vi "Actor Core.vi"(8 "error in":errorcluster, 11 "My Application":refnum<class "App Actor.lvclass">) -> (0 "error out":errorcluster, 3 "Actor out":refnum<class "Actor.lvclass">)   [LabVIEW 2024, in "App Actor.lvlib" / "App Actor.lvclass"]
doc: "This is Actor Core.vi, the main message handling loop for Actors. An actor usually just sits in this loop and processes messages as they arrive. Any error returned by the message Do.vi call will stop the loop, with error code 43 as the canonical signal to stop with no error sent to caller. Descendants may override that in Handle Error.vi."
uses:
  App Actor.lvclass
  C:/Program Files (x86)/National Instruments/LabVIEW 2024/vi.lib/ActorFramework/Actor/Actor.lvclass
  <vilib>/ActorFramework/Actor/Actor.lvclass
  HAL Interface Actor/HAL Interface Actor/HAL Interface Actor.lvclass
  DAQ Actor/DAQ Actor/DAQ Actor.lvclass
  <vilib>/ActorFramework/Actor/Actor.lvclass/Actor.ctl
  <vilib>/ActorFramework/Message Enqueuer/Message Enqueuer.lvclass/Message Enqueuer.ctl
  App Actor.lvclass/App Actor.ctl
  DAQ Actor/DAQ Actor Task Msg/DAQ Actor Task Msg.lvclass/DAQ Actor Task Msg.ctl
  HAL Interface Actor/HAL Interface Actor Task Msg/HAL Interface Actor Task Msg.lvclass/HAL Interface Actor Task Msg.ctl
  <vilib>/ActorFramework/Message Enqueuer/Init from Existing Queue.vi
  <vilib>/ActorFramework/Message Enqueuer/Enqueue.vi
  <vilib>/ActorFramework/Stop Msg/Stop Msg.lvclass
  C:/Program Files (x86)/National Instruments/LabVIEW 2024/vi.lib/ActorFramework/Message/Message.lvclass
  DAQ Actor/DAQ Actor Task Msg/DAQ Actor Task Msg.lvclass
  HAL Interface Actor/HAL Interface Actor Task Msg/HAL Interface Actor Task Msg.lvclass
  <vilib>/ActorFramework/Message Priority Queue/Priority Enqueue.vi
  <vilib>/ActorFramework/Message Enqueuer/Message Enqueuer.lvclass
panel:
  in  "stop signal":bool
  out "Event Log":string
  in  "Stop":bool
  in  "Message to DAQ Actor":bool
  in  "Message to HAL Interface Actor":bool
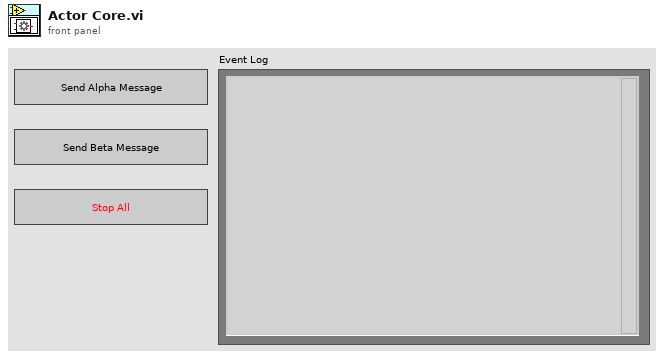
[diagram p1: front panel]
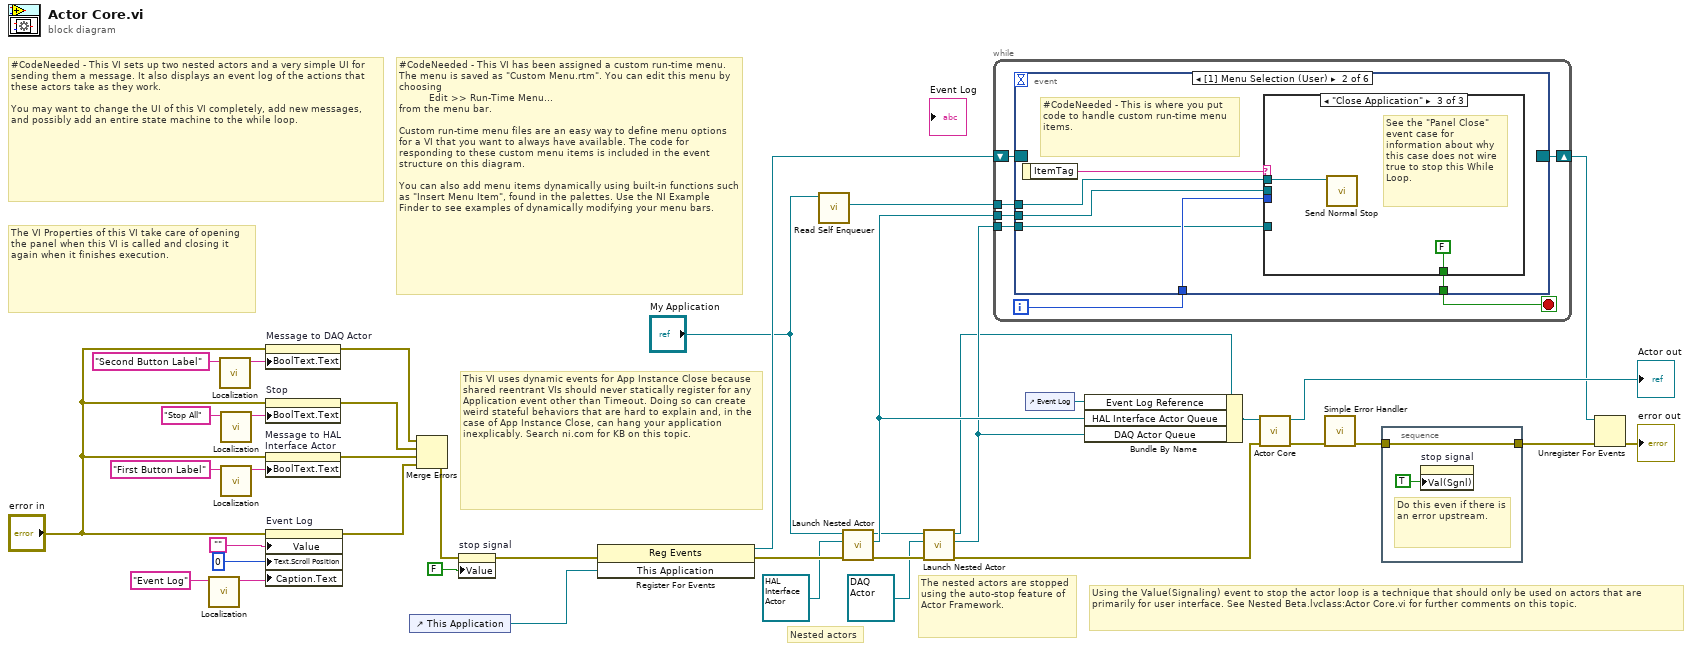
[diagram p0: block diagram]
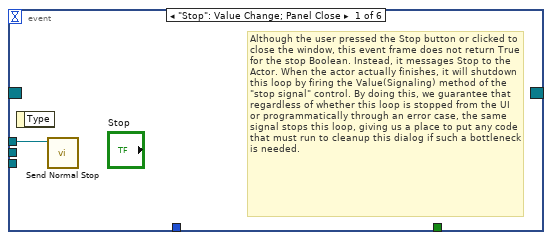
[diagram p2: hidden frame]
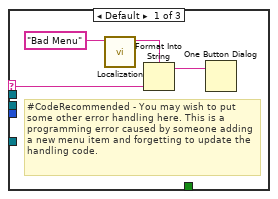
[diagram p3: hidden frame]
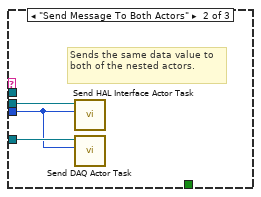
[diagram p4: hidden frame]
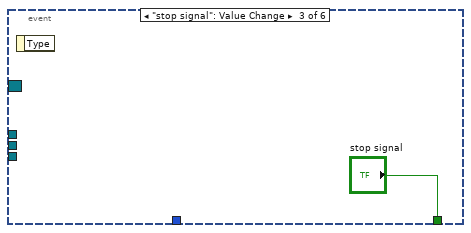
[diagram p5: hidden frame]
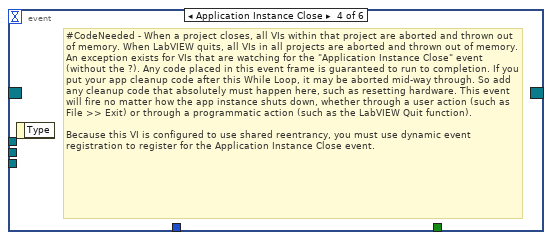
[diagram p6: hidden frame]
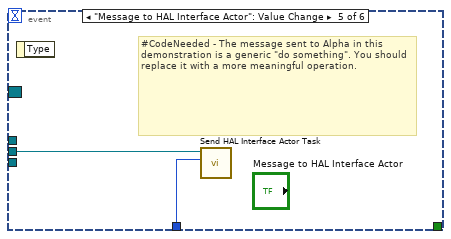
[diagram p7: hidden frame]
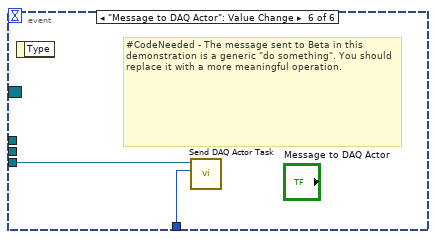
[diagram p8: hidden frame]
diagram:
  # "Nested actors"
  # "The nested actors are stopped using the auto-stop feature of Actor Framework."
  # "#CodeNeeded - This VI has been assigned a custom run-time menu. The menu is saved as \"Custom Menu.rtm\". You can edit this menu by choosing \n          Edit >> Run-Time Menu...\nfrom the menu bar.\n\nCustom run-time menu files are an easy way to define menu options for a VI that you want to always have available. The code for responding to these custom menu items is included in the event structure on this diagram.\n\nYou can also add menu items dynamically using built-in functions such as \"Insert Menu Item\", found in the palettes. Use the NI Example Finder to see examples of dynamically modifying your menu bars."
  # "This VI uses dynamic events for App Instance Close because shared reentrant VIs should never statically register for any Application event other than Timeout. Doing so can create weird stateful behaviors that are hard to explain and, in the case of App Instance Close, can hang your application inexplicably. Search ni.com for KB on this topic."
  # "The VI Properties of this VI take care of opening the panel when this VI is called and closing it again when it finishes execution."
  # "Using the Value(Signaling) event to stop the actor loop is a technique that should only be used on actors that are primarily for user interface. See Nested Beta.lvclass:Actor Core.vi for further comments on this topic."
  # "#CodeNeeded - This VI sets up two nested actors and a very simple UI for sending them a message. It also displays an event log of the actions that these actors take as they work. \n\nYou may want to change the UI of this VI completely, add new messages, and possibly add an entire state machine to the while loop."
  n1 = call "Localization.vi"("Unlocalized"="Event Log") -> ("Localized"=w26:string)  [unwired: 10 in]
  n2 = call "Localization.vi"("Unlocalized"="Second Button Label") -> ("Localized"=w20:string)  [unwired: 10 in]
  n3 = call "Localization.vi"("Unlocalized"="Stop All") -> ("Localized"=w22:string)  [unwired: 10 in]
  n4 = call "Localization.vi"("Unlocalized"="First Button Label") -> ("Localized"=w24:string)  [unwired: 10 in]
  n5 = property on="Message to DAQ Actor" class="Bool"(error in="error in", "BoolText.Text"=w20) -> (error out=w19:errorcluster)  [unwired: 1 in, 1 out]
  n6 = property on="Stop" class="Bool"(error in="error in", "BoolText.Text"=w22) -> (error out=w18:errorcluster)  [unwired: 1 in, 1 out]
  n7 = property on="Message to HAL Interface Actor" class="Bool"(error in="error in", "BoolText.Text"=w24) -> (error out=w17:errorcluster)  [unwired: 1 in, 1 out]
  n8 = property on="Event Log" class="Str"(error in="error in", "Value"="", "Text.Scroll Position"=u32 0, "Caption.Text"=w26) -> (error out=w16:errorcluster)  [unwired: 1 in, 1 out]
  n9 = control-ref of="This Application"() -> (w6:refnum<vi>)
  n10 = Merge Errors(w19, w18, w17, w16) -> (w15:errorcluster)
  n11 = property on="stop signal" class="Bool (strict)"(error in=w15, "Value"=FALSE ("stop")) -> (error out=w8:errorcluster)  [unwired: 1 in, 1 out]
  n12 = register-events(error in=w8, w6) -> (reference out=w12:refnum<event-registration>, error out=w7:errorcluster)  [unwired: 1 in]
  n13 = call <vilib>:"Read Self Enqueuer.vi"("Actor"="My Application") -> ("Self Enqueuer"=w34:refnum<class "Message Enqueuer.lvclass">)  [unwired: 10 in]
  n14 = call <vilib>:"Launch Nested Actor.vi"("error in (no error)"=w7, "Nested Actor"=refnum<class "HAL Interface Actor.lvclass"> refnum ("Alpha.lvclass"), "Caller Actor in"="My Application") -> ("error out"=w38:errorcluster, "Nested Actor's Enqueuer"=w33:refnum<class "Message Enqueuer.lvclass">, "Caller Actor out"=w4:refnum<class "App Actor.lvclass">)  [unwired: 6 in]
  n15 = call <vilib>:"Launch Nested Actor.vi"("error in (no error)"=w38, "Nested Actor"=refnum<class "DAQ Actor.lvclass"> refnum ("Beta.lvclass"), "Caller Actor in"=w4) -> ("error out"=w37:errorcluster, "Nested Actor's Enqueuer"=w32:refnum<class "Message Enqueuer.lvclass">, "Caller Actor out"=w1:refnum<class "App Actor.lvclass">)  [unwired: 6 in]
  n16 = while {
    tunnel: w34 -> [w46]
    tunnel: w33 -> [w45]
    tunnel: w32 -> [w44]
    shift-right: [w40] -> w11
    shift-left: w12 -> [w41]
    i -> [w42]
    stop <- w43 stop-if-true
    n17 = event shown="[1] Menu Selection (User)" {
      selector: w41 -> [_ _ _ _ _ _]
      dyn-events: [_ _ _ _ _ _] -> w40
      timeout: _ -> [_ _ _ _ _ _]
      tunnel: w46 -> [w47 w49 _ _ _ _]
      tunnel: w45 -> [_ w52 _ _ w65 _]
      tunnel: w44 -> [_ w50 _ _ _ w67]
      tunnel: [_ w48 "stop signal" _ _ _] -> w43
      tunnel: w42 -> [_ w51 _ _ w64 w66]
      event "Stop": Value Change; Panel Close {
        # "Although the user pressed the Stop button or clicked to close the window, this event frame does not return True for the stop Boolean. Instead, it messages Stop to the Actor. When the actor actually finishes, it will shutdown this loop by firing the Value(Signaling) method of the \"stop signal\" control. By doing this, we guarantee that regardless of whether this loop is stopped from the UI or programmatically through an error case, the same signal stops this loop, giving us a place to put any code that must run to cleanup this dialog if such a bottleneck is needed."
        n18 = event-data() -> ()  [unwired: 1 in, 1 out]
        n19 = call <vilib>:"Send Normal Stop.vi"("Message Enqueuer"=w47) -> ()  [unwired: 10 in, 1 out]
      }
      event Menu Selection (User) {
        # "#CodeNeeded - This is where you put code to handle custom run-time menu items."
        n20 = event-data() -> ("ItemTag"=w53:string)  [unwired: 1 in]
        n21 = case shown="\"Close Application\"" w53 {
          selector: w53 -> [w55 _ _]
          tunnel: w52 -> [_ w60 _]
          tunnel: w51 -> [_ w58 _]
          tunnel: w50 -> [_ w59 _]
          tunnel: w49 -> [_ _ w62]
          tunnel: [_ _ FALSE] -> w48
          frame Default {
            # "#CodeRecommended - You may wish to put some other error handling here. This is a programming error caused by someone adding a new menu item and forgetting to update the handling code."
            n22 = call "Localization.vi"("Unlocalized"="Bad Menu") -> ("Localized"=w56:string)  [unwired: 10 in]
            n23 = Format Into String(format string=w56, w55) -> (resulting string=w54:string)  [unwired: 2 in, 1 out]
            n24 = One Button Dialog(message=w54) -> ()  [unwired: 1 in, 1 out]
          }
          frame "Send Message To Both Actors" {
            # "Sends the same data value to both of the nested actors."
            n25 = call "Send HAL Interface Actor Task.vi"("Data"=w58, "Message Enqueuer"=w60) -> ()  [unwired: 9 in, 1 out]
            n26 = call "Send DAQ Actor Task.vi"("Data"=w58, "Message Enqueuer"=w59) -> ()  [unwired: 9 in, 1 out]
          }
          frame "Close Application" {
            # "See the \"Panel Close\" event case for information about why this case does not wire true to stop this While Loop."
            n27 = call <vilib>:"Send Normal Stop.vi"("Message Enqueuer"=w62) -> ()  [unwired: 10 in, 1 out]
          }
        }
      }
      event "stop signal": Value Change {
        n28 = event-data() -> ()  [unwired: 1 in, 1 out]
      }
      event Application Instance Close {
        # "#CodeNeeded - When a project closes, all VIs within that project are aborted and thrown out of memory. When LabVIEW quits, all VIs in all projects are aborted and thrown out of memory. An exception exists for VIs that are watching for the \"Application Instance Close\" event (without the ?). Any code placed in this event frame is guaranteed to run to completion. If you put your app cleanup code after this While Loop, it may be aborted mid-way through. So add any cleanup code that absolutely must happen here, such as resetting hardware. This event will fire no matter how the app instance shuts down, whether through a user action (such as File >> Exit) or through a programmatic action (such as the LabVIEW Quit function).\n\nBecause this VI is configured to use shared reentrancy, you must use dynamic event registration to register for the Application Instance Close event."
        n29 = event-data() -> ()  [unwired: 1 in, 1 out]
      }
      event "Message to HAL Interface Actor": Value Change {
        # "#CodeNeeded - The message sent to Alpha in this demonstration is a generic \"do something\". You should replace it with a more meaningful operation."
        n30 = event-data() -> ()  [unwired: 1 in, 1 out]
        n31 = call "Send HAL Interface Actor Task.vi"("Data"=w64, "Message Enqueuer"=w65) -> ()  [unwired: 9 in, 1 out]
      }
      event "Message to DAQ Actor": Value Change {
        # "#CodeNeeded - The message sent to Beta in this demonstration is a generic \"do something\". You should replace it with a more meaningful operation."
        n32 = event-data() -> ()  [unwired: 1 in, 1 out]
        n33 = call "Send DAQ Actor Task.vi"("Data"=w66, "Message Enqueuer"=w67) -> ()  [unwired: 9 in, 1 out]
      }
    }
  }
  n34 = control-ref of="Event Log"() -> (w35:refnum<vi>)
  n35 = Bundle By Name(cluster=w1, "Event Log Reference"=w35, "HAL Interface Actor Queue"=w33, "DAQ Actor Queue"=w32) -> (w36:refnum<class "App Actor.lvclass">)
  n36 = call-parent "Actor Core.vi"("error in"=w37, "Actor in"=w36) -> ("error out"=w14:errorcluster, "Actor out"=→"Actor out":refnum<class "Actor.lvclass">)  [unwired: 8 in]
  n37 = call <vilib>:"Simple Error Handler.vi"("error in (no error)"=w14) -> ("error out"=w13:errorcluster)  [unwired: 4 in, 4 out]
  n38 = stacked-sequence {
    tunnel: [w68] -> w10
    tunnel: w13 -> [w68]
    frame #0 {
      # "Do this even if there is an error upstream."
      n39 = property on="stop signal" class="Bool (strict)"("Val(Sgnl)"=TRUE ("stop")) -> ()  [unwired: 2 in, 2 out]
    }
  }
  n40 = Unregister For Events(event registration refnum=w11, error in=w10) -> (error out=→"error out":errorcluster)
